vi "VI Tree.vi"   [LabVIEW 2015, in "Chroma ATE 6310.lvlib"]
doc: "This is the instrument driver for the CHROMA 6310 Programmable DC Electronic Load. The VI Tree displays all the user-callable VIs of the instrument driver in an organized table."
uses:
  <instrlib>/Chroma ATE 6310/Chroma ATE 6310.lvlib
panel:
  # "© 2005 National Instruments.  ALL RIGHTS RESERVED."
  # "See the diagram\nFor the VI Tree"
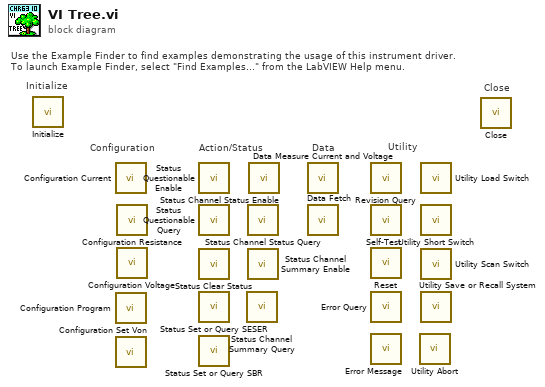
[diagram p0: block diagram]
diagram:
  # "Data"
  # "Use the Example Finder to find examples demonstrating the usage of this instrument driver.\nTo launch Example Finder, select \"Find Examples...\" from the LabVIEW Help menu."
  # "Initialize"
  # "Configuration"
  # "Utility"
  # "Action/Status"
  # "Close"
  n1 = call <instrlib>:"Initialize.vi"() -> ()  [unwired: 10 in, 2 out]
  n2 = call <instrlib>:"Configuration Current.vi"() -> ()  [unwired: 18 in, 2 out]
  n3 = call <instrlib>:"Configuration Program.vi"() -> ()  [unwired: 18 in, 2 out]
  n4 = call <instrlib>:"Configuration Set Von.vi"() -> ()  [unwired: 14 in, 2 out]
  n5 = call <instrlib>:"Configuration Resistance.vi"() -> ()  [unwired: 14 in, 2 out]
  n6 = call <instrlib>:"Configuration Voltage.vi"() -> ()  [unwired: 14 in, 2 out]
  n7 = call <instrlib>:"Status Questionable Enable.vi"() -> ()  [unwired: 14 in, 2 out]
  n8 = call <instrlib>:"Status Questionable Query.vi"() -> ()  [unwired: 13 in, 3 out]
  n9 = call <instrlib>:"Status Clear Status.vi"() -> ()  [unwired: 14 in, 2 out]
  n10 = call <instrlib>:"Status Set or Query SESER.vi"() -> ()  [unwired: 13 in, 3 out]
  n11 = call <instrlib>:"Status Set or Query SBR.vi"() -> ()  [unwired: 13 in, 3 out]
  n12 = call <instrlib>:"Status Channel Summary Query.vi"() -> ()  [unwired: 13 in, 3 out]
  n13 = call <instrlib>:"Status Channel Status Query.vi"() -> ()  [unwired: 13 in, 3 out]
  n14 = call <instrlib>:"Status Channel Summary Enable.vi"() -> ()  [unwired: 14 in, 2 out]
  n15 = call <instrlib>:"Status Channel Status Enable.vi"() -> ()  [unwired: 14 in, 2 out]
  n16 = call <instrlib>:"Data Measure Current and Voltage.vi"() -> ()  [unwired: 12 in, 4 out]
  n17 = call <instrlib>:"Data Fetch.vi"() -> ()  [unwired: 11 in, 5 out]
  n18 = call <instrlib>:"Revision Query.vi"() -> ()  [unwired: 12 in, 4 out]
  n19 = call <instrlib>:"Self-Test.vi"() -> ()  [unwired: 12 in, 4 out]
  n20 = call <instrlib>:"Reset.vi"() -> ()  [unwired: 14 in, 2 out]
  n21 = call <instrlib>:"Error Query.vi"() -> ()  [unwired: 12 in, 4 out]
  n22 = call <instrlib>:"Error Message.vi"() -> ()  [unwired: 11 in, 5 out]
  n23 = call <instrlib>:"Utility Abort.vi"() -> ()  [unwired: 14 in, 2 out]
  n24 = call <instrlib>:"Utility Load Switch.vi"() -> ()  [unwired: 14 in, 2 out]
  n25 = call <instrlib>:"Utility Short Switch.vi"() -> ()  [unwired: 14 in, 2 out]
  n26 = call <instrlib>:"Utility Scan Switch.vi"() -> ()  [unwired: 14 in, 2 out]
  n27 = call <instrlib>:"Utility Save or Recall System.vi"() -> ()  [unwired: 14 in, 2 out]
  n28 = call <instrlib>:"Close.vi"() -> ()  [unwired: 15 in, 1 out]
